vi "Keithley J-t List_IIT.vi"(0 "VISA resource name in":refnum<visa-resource-name>, 11 "Voltage List":dbl[](array[numeric])) -> (4 "VISA resource name out":refnum<visa-resource-name>, 6 "Data Array":dbl[][](array[numeric]), 15 "Measurement Complete":bool)   [LabVIEW 2011]
doc: "Configures a sweep and takes voltage and current readings at each point."
uses:
  <instrlib>/keithley_24xx/Keithley 24XX/Public/Data/Read (Multiple Points).vi
  <instrlib>/keithley_24xx/Keithley 24XX/Keithley 24XX.lvlib
panel:
  in  "Source Mode  (0: Voltage)":u16(ring) items=["Voltage", "Current"]
  # "(c) 2006 National Instruments.  ALL RIGHTS RESERVED."
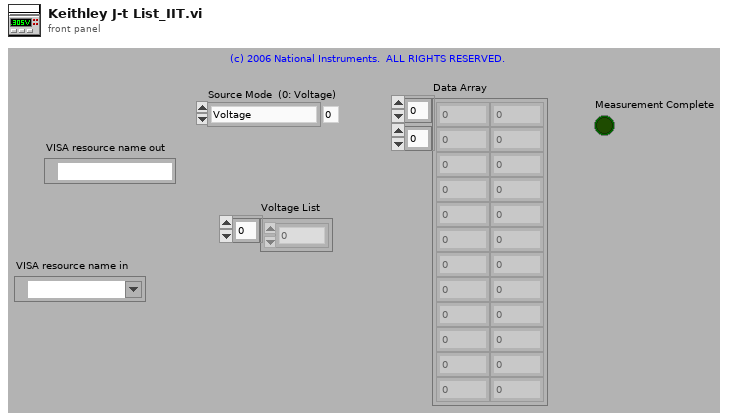
[diagram p1: front panel]
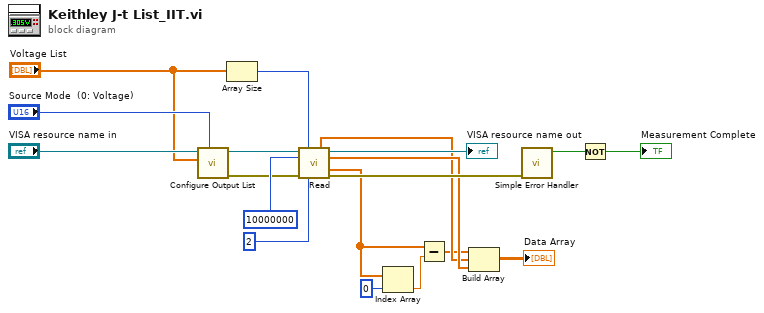
[diagram p0: block diagram]
diagram:
  n1 = call <instrlib>:"Configure Output List.vi"("Source Mode  (0: Voltage)"="Source Mode  (0: Voltage)", "Output List"="Voltage List", "VISA resource name"="VISA resource name in") -> ("error out"=w11:errorcluster, "VISA resource name out"=w12:refnum<visa-resource-name>)  [unwired: 7 in]
  n2 = Array Size(array="Voltage List") -> (size(s)=w6:i32)
  n3 = call-poly <instrlib>:"Read.vi"("VISA resource name"=w12, "Sample Count (1)"=w6, "Timeout (10000 ms)"=10000000, "error in (no error)"=w11, "Output Mode (0: Fixed)"=2) -> ("Voltage"=w5:sgl[], "VISA resource name out"=→"VISA resource name out":refnum<visa-resource-name>, "Current"=w8:sgl[], "Timestamp"=w2:sgl[], "error out"=w19:errorcluster)  [unwired: 4 in, 2 out]
  n4 = Index Array(array=w2, index=0) -> (element=w4:sgl)
  n5 = Subtract(x=w2, y=w4) -> (x-y=w3:sgl[])
  n6 = Build Array(w3, w5, w8) -> (→"Data Array":sgl[][])
  n7 = call <vilib>:"Simple Error Handler.vi"("error in (no error)"=w19) -> ("error?"=w17:bool)  [unwired: 4 in, 4 out]
  n8 = Not(x=w17) -> (.not. x?=→"Measurement Complete":bool)
